vi "Read Channel Configurations from Listbox.vi"(8 "error in":errorcluster, 11 "MulticolumnListbox in":refnum<vi>) -> (0 "error out":errorcluster, 2 "Plot Channel Configurations":T1[](array[typedef]))   [LabVIEW 2017, in "DTacq Plot Display Library.lvlib"]
uses:
  DTacq Plot Display Library.lvlib
  Typedefs/Plot Channel Configruation--Cluster.ctl
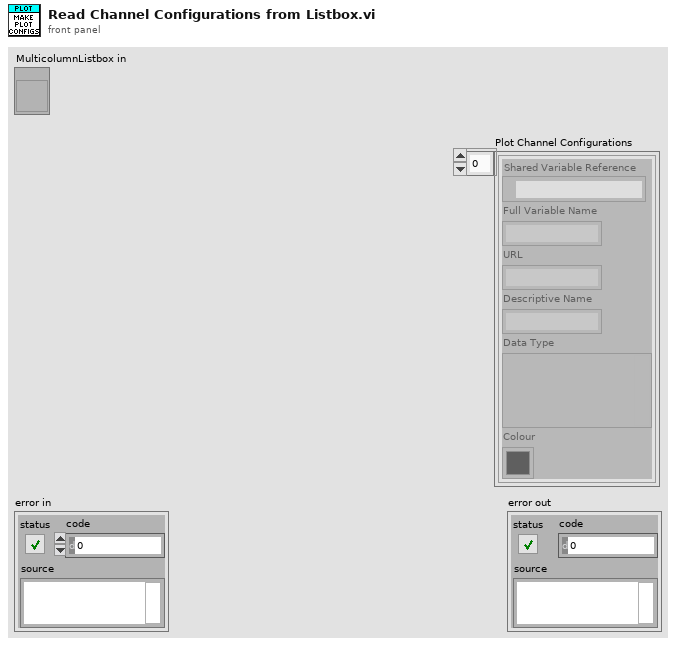
[diagram p1: front panel]
types:
  T1 = typedef "DTacq Plot Display Library.lvlib/Plot Channel Configruation--Cluster.ctl" = cluster{"Shared Variable Reference":refnum<k21>, "Full Variable Name":string, "URL":string, "Descriptive Name":string, "Data Type":variant, "Colour":u32}
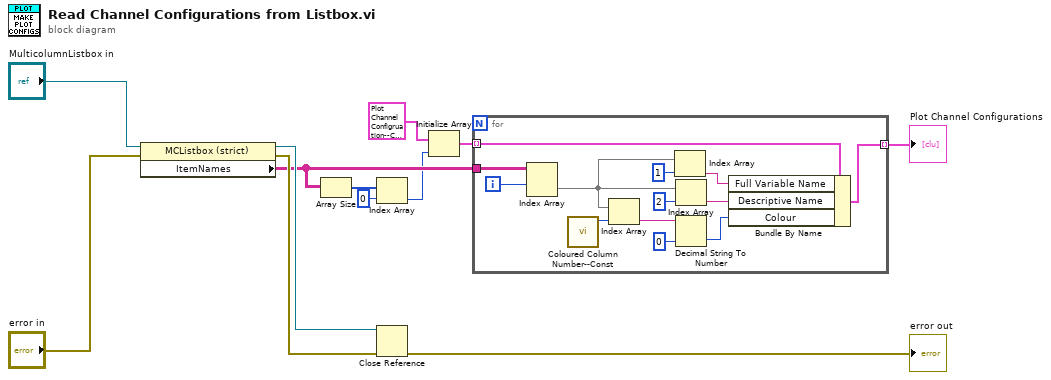
[diagram p0: block diagram]
diagram:
  n1 = property class="MCListbox (strict)"(reference="MulticolumnListbox in", error in="error in") -> (reference out=w8:refnum<vi>, error out=w7:errorcluster, "ItemNames"=w3:string[][])
  n2 = Array Size(array=w3) -> (size(s)=w4:i32[])
  n3 = Index Array(array=w4, index=0) -> (element=w1:i32)
  n4 = Close Reference(reference=w8, error in (no error)=w7) -> (error out=→"error out":errorcluster)
  n5 = Initialize Array(T1 {"Shared Variable Reference"="", "Full Variable Name"="", "URL"="", "Descriptive Name"="", "Data Type"=variant, "Colour"=0} ("Plot Channel Configuration"), w1) -> (w10:T1[])
  n6 = for {
    tunnel: w10 -> [w22] mode=indexing
    tunnel: w3 -> [w25]
    tunnel: [w14] -> w5 mode=indexing
    i -> [w24]
    n7 = Index Array(array=w25, index (row)=w24) -> (element=w16:string[])  [unwired: 1 in]
    n8 = call "Coloured Column Number--Const.vi"() -> ("Coloured Column"=w23:i32)  [unwired: 11 in]
    n9 = Index Array(array=w16, index=w23) -> (element=w21:string)
    n10 = Index Array(array=w16, index=1) -> (element=w15:string)
    n11 = Index Array(array=w16, index=2) -> (element=w17:string)
    n12 = Decimal String To Number(string=w21, default (0L)=u32 0 ("Colour")) -> (number=w19:u32)  [unwired: 1 in, 1 out]
    n13 = Bundle By Name(cluster=w22, "Full Variable Name"=w15, "Descriptive Name"=w17, "Colour"=w19) -> (w14:T1)
  }
  "Plot Channel Configurations" <- w5
